vi "Format into Table.vi"(8 "error in (no error)":errorcluster, 11 "Expense Summary in":refnum<class "Expense Summary.lvclass">) -> (0 "error out":errorcluster, 2 "Summary Values":string[](array[string]), 3 "Expense Summary out":refnum<class "Expense Summary.lvclass">)   [LabVIEW 2018, in "Expense Summary.lvclass"]
uses:
  Expense Summary.lvclass
  Expense Summary.lvclass/Expense Summary.ctl
  Category/Category.lvclass
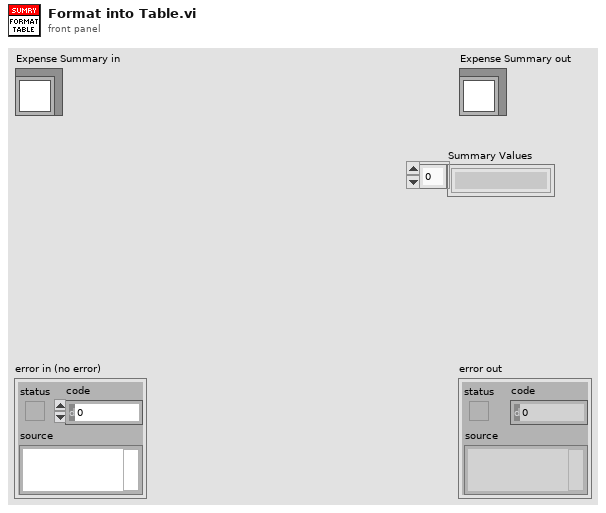
[diagram p1: front panel]
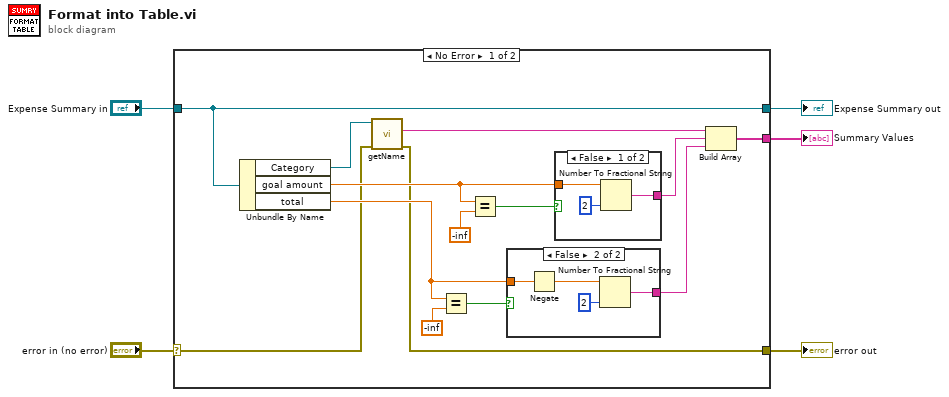
[diagram p0: block diagram]
diagram:
  n1 = case shown="No Error" "error in (no error)" {
    selector: "error in (no error)" -> [w9 w28]
    tunnel: [w8 w28] -> w4
    tunnel: [w19 w27] -> w2
    tunnel: "Expense Summary in" -> [w19 w27]
    tunnel: [w12 _] -> w1
    frame No Error {
      n2 = Unbundle By Name(w19) -> ("Category"=w7:refnum<class "Category.lvclass">, "goal amount"=w15:dbl, "total"=w17:dbl)
      n3 = call "getName.vi"("error in (no error)"=w9, "Category in"=w7) -> ("error out"=w8:errorcluster, "Name"=w6:string)  [unwired: 7 in, 1 out]
      n4 = Equal?(x=w17, y=-inf) -> (x = y?=w18:bool)
      n5 = Equal?(x=w15, y=-inf) -> (x = y?=w16:bool)
      n6 = case shown="False" w18 {
        tunnel: w17 -> [_ w24]
        tunnel: [_ w25] -> w13
        frame True {
        }
        frame False {
          n7 = Negate(x=w24) -> (-x=w23:dbl)
          n8 = Number To Fractional String(number=w23, precision (6)=i16 2) -> (F-format string=w25:string)  [unwired: 2 in]
        }
      }
      n9 = case shown="False" w16 {
        tunnel: w15 -> [w21 _]
        tunnel: [w20 _] -> w14
        frame False {
          n10 = Number To Fractional String(number=w21, precision (6)=i16 2) -> (F-format string=w20:string)  [unwired: 2 in]
        }
        frame True {
        }
      }
      n11 = Build Array(w6, w14, w13) -> (w12:string[])
    }
    frame Error {
    }
  }
  "error out" <- w4
  "Expense Summary out" <- w2
  "Summary Values" <- w1
